vi "Save_to_Project.vi"(8 "error in (no error)":errorcluster, 11 "AB_Build in":refnum<class "AB_Build.lvclass">) -> (0 "error out":errorcluster, 3 "AB_Build out":refnum<class "AB_Build.lvclass">)   [LabVIEW 2020, in "AB_Build.lvclass"]
uses:
  <vilib>/AppBuilder/AB_Classes/Build/AB_Build.lvclass
  <vilib>/AppBuilder/AB_Classes/Build/AB_Build.lvclass/AB_Build.ctl
  <vilib>/AppBuilder/RW_Project/AB_RW_Project_PropBag_Action.ctl
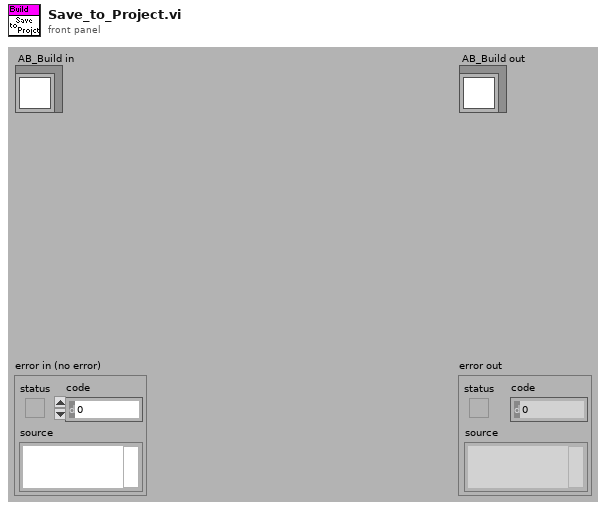
[diagram p1: front panel]
types:
  T1 = typedef "AB_RW_Project_PropBag_Action.ctl" = enum16{"read", "write", "clear", "readPrevious", "writePrevious", "clearPrevious"}
  T2 = typedef "ItemRef.ctl" = u64
  T3 = typedef "AB_RW_Non_Persistent_Data.ctl" = cluster{"AB_Class_Path":path, "AB_UIClass_Path":path}
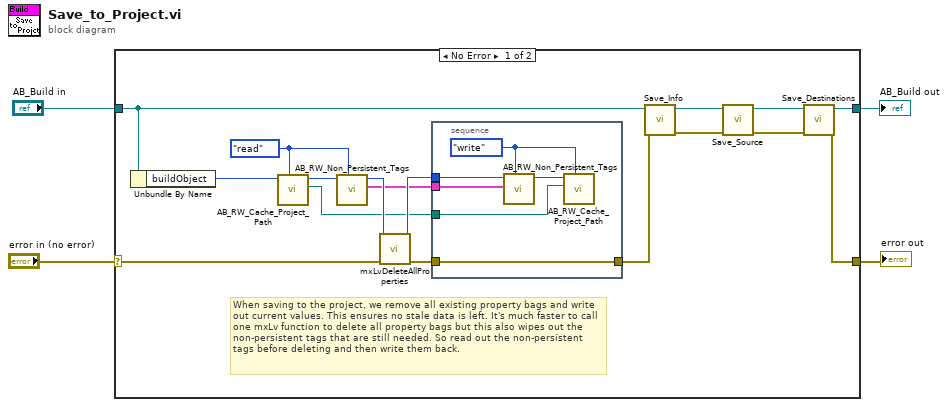
[diagram p0: block diagram]
diagram:
  n1 = case shown="No Error" "error in (no error)" {
    selector: "error in (no error)" -> [w13 w29]
    tunnel: [w16 w29] -> w3
    tunnel: [w19 w28] -> w1
    tunnel: "AB_Build in" -> [w15 w28]
    frame No Error {
      w8 = AB_RW_Project_PropBag_Action."read" ("action")
      # "When saving to the project, we remove all existing property bags and write out current values. This ensures no stale data is left. It's much faster to call one mxLv function to delete all property bags but this also wipes out the non-persistent tags that are still needed. So read out the non-persistent tags before deleting and then write them back."
      n2 = Unbundle By Name(w15) -> ("buildObject"=w7:T2)
      n3 = call <vilib>:"AB_RW_Cache_Project_Path.vi"("action"=w8, "buildObject"=w7) -> ("ProjectPath out"=w5:path, "buildObject out"=w6:T2)  [unwired: 7 in, 1 out]
      n4 = call <vilib>:"AB_RW_Non_Persistent_Tags.vi"("action"=w8, "buildObject"=w6) -> ("data out"=w11:T3, "buildObject out"=w14:T2)  [unwired: 7 in, 1 out]
      n5 = call <resource>:"mxLvDeleteAllProperties.vi"("error in"=w13, "Item"=w14) -> ("error out"=w10:errorcluster, "Item"=w12:T2)  [unwired: 8 in]
      n6 = stacked-sequence {
        tunnel: w12 -> [w27]
        tunnel: w11 -> [w26]
        tunnel: w10 -> [w25]
        tunnel: [w25] -> w9
        tunnel: w5 -> [w22]
        frame #0 {
          w23 = AB_RW_Project_PropBag_Action."write" ("action")
          n7 = call <vilib>:"AB_RW_Non_Persistent_Tags.vi"("action"=w23, "data in"=w26, "buildObject"=w27) -> ("buildObject out"=w24:T2)  [unwired: 6 in, 2 out]
          n8 = call <vilib>:"AB_RW_Cache_Project_Path.vi"("action"=w23, "ProjectPath in"=w22, "buildObject"=w24) -> ()  [unwired: 6 in, 3 out]
        }
      }
      n9 = call-dynamic "Save_Info.vi"("error in (no error)"=w9, "AB_Build in"=w15) -> ("error out"=w18:errorcluster, "AB_Build out"=w21:refnum<class "AB_Build.lvclass">)  [unwired: 8 in]
      n10 = call-dynamic "Save_Source.vi"("error in (no error)"=w18, "AB_Build in"=w21) -> ("error out"=w17:errorcluster, "AB_Build out"=w20:refnum<class "AB_Build.lvclass">)  [unwired: 8 in]
      n11 = call-dynamic "Save_Destinations.vi"("error in (no error)"=w17, "AB_Build in"=w20) -> ("error out"=w16:errorcluster, "AB_Build out"=w19:refnum<class "AB_Build.lvclass">)  [unwired: 8 in]
    }
    frame Error {
    }
  }
  "error out" <- w3
  "AB_Build out" <- w1
